vi "CANOpen_SetGet Bus Settings.vi"(6 "Set Parameters":bool, 8 "error in (no error)":errorcluster, 10 "Parameters":variant, 11 "CANOpen Bus Settings":T1={"CANOpen Interface Name"=0, "Baud Rate"=0, "Termination"=FALSE, "Sync Period (ms)"=10, "Enable 9881"=FALSE, "RIO Device"=0, "Enable SYNC"=FALSE, "Scan & Print"=FALSE} {"Baud Rate" items=["1 Mbit/s"=0, "800 kbit/s"=1, "500 kbit/s"=2, "250 kbit/s"=3, "125 kbit/s"=4, "50 kbit/s"=6, "20 kbit/s"=7, "10 kbit/s"=8]; "CANOpen Interface Name" items=["CANopen01", "CANopen02", "CANopen03", "CANopen04", "CANopen05", "CANopen06", "CANopen07", "CANopen08", "CANopen09", "CANopen10", "CANopen11", "CANopen12", "CANopen13", "CANopen14", "CANopen15", "CANopen16", "CANopen17", "CANopen18", "CANopen19", "CANopen20", "CANopen21", "CANopen22", "CANopen23", "CANopen24", "CANopen25", "CANopen26", "CANopen27", "CANopen28", "CANopen29", "CANopen30", "CANopen31", "CANopen32"]}) -> (0 "error out":errorcluster, 2 "Parameters":variant, 3 "CANOpen Bus Settings":T1={"CANOpen Interface Name"=0, "Baud Rate"=0, "Termination"=FALSE, "Sync Period (ms)"=10, "Enable 9881"=FALSE, "RIO Device"=0, "Enable SYNC"=FALSE, "Scan & Print"=FALSE} {"Baud Rate" items=["1 Mbit/s"=0, "800 kbit/s"=1, "500 kbit/s"=2, "250 kbit/s"=3, "125 kbit/s"=4, "50 kbit/s"=6, "20 kbit/s"=7, "10 kbit/s"=8]; "CANOpen Interface Name" items=["CANopen01", "CANopen02", "CANopen03", "CANopen04", "CANopen05", "CANopen06", "CANopen07", "CANopen08", "CANopen09", "CANopen10", "CANopen11", "CANopen12", "CANopen13", "CANopen14", "CANopen15", "CANopen16", "CANopen17", "CANopen18", "CANopen19", "CANopen20", "CANopen21", "CANopen22", "CANopen23", "CANopen24", "CANopen25", "CANopen26", "CANopen27", "CANopen28", "CANopen29", "CANopen30", "CANopen31", "CANopen32"]})   [LabVIEW 2021, in "CANOpen Addon Engine.lvlib"]
uses:
  CANOpen Addon Engine.lvlib
  Shared/CANOpen_Bus Settings.ctl
  Shared/CANOpen Interface Name.ctl
  <vilib>/CANopenLib/CANOPEN.llb/CANopen BaudRate.ctl
  Shared/CANOpen Addon GUID Lookup Global.vi
  Shared/CANOpen Addon Shared.lvlib
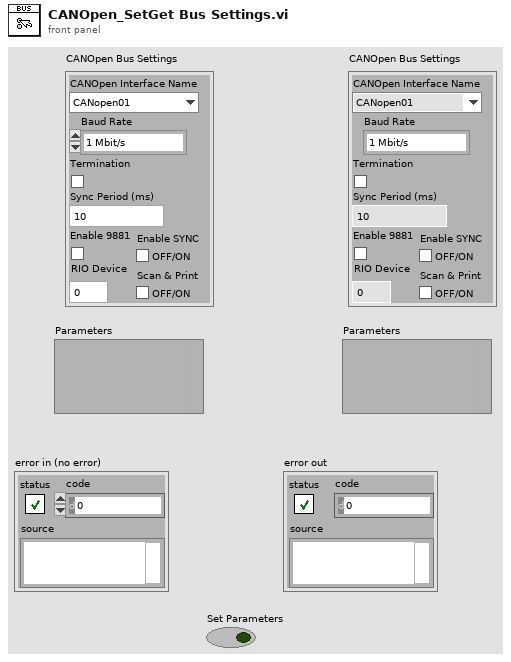
[diagram p1: front panel]
types:
  T1 = typedef "CANOpen Addon Shared.lvlib/CANOpen_Bus Settings.ctl" = cluster{"CANOpen Interface Name":T2, "Baud Rate":T3, "Termination":bool, "Sync Period (ms)":i64, "Enable 9881":bool, "RIO Device":u16, "Enable SYNC":bool, "Scan & Print":bool}
  T2 = typedef "CANOpen Addon Shared.lvlib/CANOpen Interface Name.ctl" = u32
  T3 = typedef "CANopen BaudRate.ctl" = u32
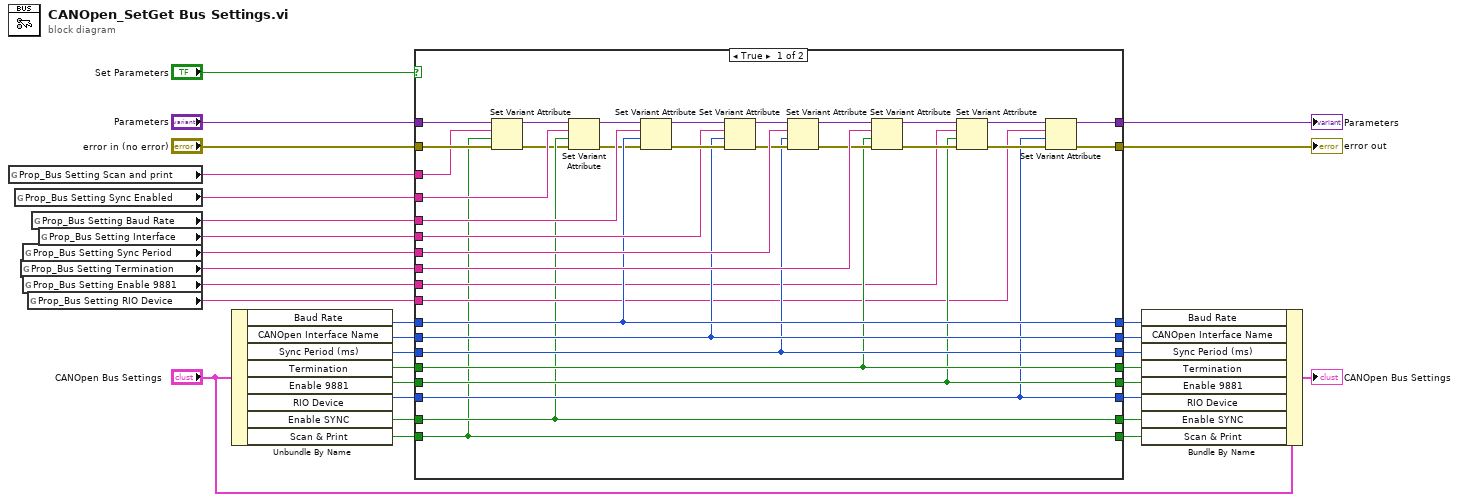
[diagram p0: block diagram]
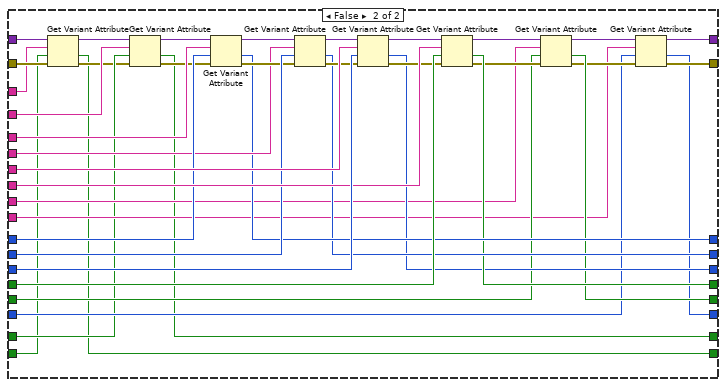
[diagram p2: hidden frame]
diagram:
  n1 = global read "CANOpen Addon GUID Lookup Global.vi" "Prop_Bus Setting Scan and print"() -> (w1:string)
  n2 = global read "CANOpen Addon GUID Lookup Global.vi" "Prop_Bus Setting Sync Enabled"() -> (w5:string)
  n3 = global read "CANOpen Addon GUID Lookup Global.vi" "Prop_Bus Setting Termination"() -> (w27:string)
  n4 = global read "CANOpen Addon GUID Lookup Global.vi" "Prop_Bus Setting Sync Period"() -> (w26:string)
  n5 = global read "CANOpen Addon GUID Lookup Global.vi" "Prop_Bus Setting Enable 9881"() -> (w13:string)
  n6 = global read "CANOpen Addon GUID Lookup Global.vi" "Prop_Bus Setting RIO Device"() -> (w8:string)
  n7 = global read "CANOpen Addon GUID Lookup Global.vi" "Prop_Bus Setting Baud Rate"() -> (w21:string)
  n8 = global read "CANOpen Addon GUID Lookup Global.vi" "Prop_Bus Setting Interface"() -> (w22:string)
  n9 = Unbundle By Name("CANOpen Bus Settings") -> ("Baud Rate"=w24:T3, "CANOpen Interface Name"=w25:T2, "Sync Period (ms)"=w28:i64, "Termination"=w29:bool, "Enable 9881"=w12:bool, "RIO Device"=w10:u16, "Enable SYNC"=w7:bool, "Scan & Print"=w3:bool)
  n10 = case shown="True" "Set Parameters" {
    tunnel: [w44 w84] -> w31
    tunnel: [w45 w83] -> w30
    tunnel: w29 -> [w52 w107]
    tunnel: w28 -> [w53 w106]
    tunnel: w27 -> [w65 w105]
    tunnel: w26 -> [w64 w104]
    tunnel: w25 -> [w54 w99]
    tunnel: w24 -> [w55 w98]
    tunnel: "error in (no error)" -> [w34 w70]
    tunnel: w22 -> [w58 w96]
    tunnel: w21 -> [w56 w94]
    tunnel: [w55 w93] -> w18
    tunnel: [w54 w92] -> w17
    tunnel: [w52 w91] -> w15
    tunnel: [w53 w90] -> w16
    tunnel: w13 -> [w49 w86]
    tunnel: w12 -> [w48 w87]
    tunnel: [w48 w85] -> w11
    tunnel: w10 -> [w43 w80]
    tunnel: [w43 w79] -> w9
    tunnel: w8 -> [w42 w81]
    tunnel: w7 -> [w38 w75]
    tunnel: [w38 w74] -> w6
    tunnel: w5 -> [w39 w73]
    tunnel: "Parameters" -> [w35 w71]
    tunnel: w3 -> [w32 w68]
    tunnel: [w32 w67] -> w2
    tunnel: w1 -> [w33 w66]
    frame True {
      n11 = Set Variant Attribute(Variant=w35, name=w33, value=w32, error in=w34) -> (Variant out=w37:variant, error out=w36:errorcluster)  [unwired: 1 out]
      n12 = Set Variant Attribute(Variant=w37, name=w39, value=w38, error in=w36) -> (Variant out=w41:variant, error out=w40:errorcluster)  [unwired: 1 out]
      n13 = Set Variant Attribute(Variant=w41, name=w56, value=w55, error in=w40) -> (Variant out=w57:variant, error out=w59:errorcluster)  [unwired: 1 out]
      n14 = Set Variant Attribute(Variant=w57, name=w58, value=w54, error in=w59) -> (Variant out=w62:variant, error out=w63:errorcluster)  [unwired: 1 out]
      n15 = Set Variant Attribute(Variant=w62, name=w64, value=w53, error in=w63) -> (Variant out=w61:variant, error out=w60:errorcluster)  [unwired: 1 out]
      n16 = Set Variant Attribute(Variant=w61, name=w65, value=w52, error in=w60) -> (Variant out=w51:variant, error out=w50:errorcluster)  [unwired: 1 out]
      n17 = Set Variant Attribute(Variant=w51, name=w49, value=w48, error in=w50) -> (Variant out=w47:variant, error out=w46:errorcluster)  [unwired: 1 out]
      n18 = Set Variant Attribute(Variant=w47, name=w42, value=w43, error in=w46) -> (Variant out=w44:variant, error out=w45:errorcluster)  [unwired: 1 out]
    }
    frame False {
      n19 = Get Variant Attribute(Variant=w71, name=w66, default value (empty Variant)=w68, error in=w70) -> (duplicate Variant=w72:variant, value=w67:bool, error out=w69:errorcluster)  [unwired: 1 out]
      n20 = Get Variant Attribute(Variant=w72, name=w73, default value (empty Variant)=w75, error in=w69) -> (duplicate Variant=w77:variant, value=w74:bool, error out=w76:errorcluster)  [unwired: 1 out]
      n21 = Get Variant Attribute(Variant=w77, name=w94, default value (empty Variant)=w98, error in=w76) -> (duplicate Variant=w95:variant, value=w93:T3, error out=w97:errorcluster)  [unwired: 1 out]
      n22 = Get Variant Attribute(Variant=w95, name=w96, default value (empty Variant)=w99, error in=w97) -> (duplicate Variant=w102:variant, value=w92:T2, error out=w103:errorcluster)  [unwired: 1 out]
      n23 = Get Variant Attribute(Variant=w102, name=w104, default value (empty Variant)=w106, error in=w103) -> (duplicate Variant=w101:variant, value=w90:i64, error out=w100:errorcluster)  [unwired: 1 out]
      n24 = Get Variant Attribute(Variant=w101, name=w105, default value (empty Variant)=w107, error in=w100) -> (duplicate Variant=w88:variant, value=w91:bool, error out=w89:errorcluster)  [unwired: 1 out]
      n25 = Get Variant Attribute(Variant=w88, name=w86, default value (empty Variant)=w87, error in=w89) -> (duplicate Variant=w78:variant, value=w85:bool, error out=w82:errorcluster)  [unwired: 1 out]
      n26 = Get Variant Attribute(Variant=w78, name=w81, default value (empty Variant)=w80, error in=w82) -> (duplicate Variant=w84:variant, value=w79:u16, error out=w83:errorcluster)  [unwired: 1 out]
    }
  }
  "Parameters" <- w31
  "error out" <- w30
  n27 = Bundle By Name(cluster="CANOpen Bus Settings", "Baud Rate"=w18, "CANOpen Interface Name"=w17, "Sync Period (ms)"=w16, "Termination"=w15, "Enable 9881"=w11, "RIO Device"=w9, "Enable SYNC"=w6, "Scan & Print"=w2) -> (→"CANOpen Bus Settings":T1)
